vi "JKI SM Editor - Search String to Search Array.vi"(1 "String":string) -> (0 "Array":string[](array[string]))   [LabVIEW 2020]
uses:
  <userlib>/_OpenG.lib/string/string.llb/Trim Whitespace (String)__ogtk.vi
  <userlib>/_OpenG.lib/string/string.llb/openg_string.lvlib
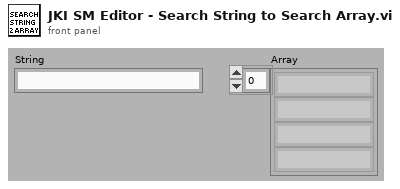
[diagram p1: front panel]
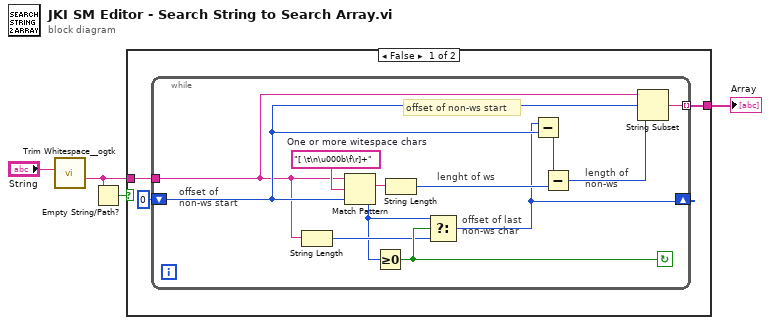
[diagram p0: block diagram]
diagram:
  n1 = call-poly <userlib>:"Trim Whitespace__ogtk.vi"("String in"="String") -> ("String out"=w2:string)  [unwired: 6 in]
  n2 = Empty String/Path?(string/path=w2) -> (empty?=w1:bool)
  n3 = case shown="False" w1 {
    tunnel: [w7 _] -> w4
    tunnel: w2 -> [w5 _]
    frame False {
      n4 = while {
        shift-right: [w8] -> _
        shift-left: 0 -> [w14]
        tunnel: w5 -> [w11]
        tunnel: [w15] -> w7 mode=indexing
        stop <- w12 continue-if-true
        w19 = "[ \t\n\u000b\f\r]+"  # One or more witespace chars
        # "offset of non-ws start"
        # "length of non-ws"
        # "offset of non-ws start"
        # "lenght of ws"
        # "offset of last non-ws char"
        n5 = String Length(string=w11) -> (length=w10:i32)
        n6 = Match Pattern(string=w11, regular expression=w19, offset (0)=w14) -> (match substring=w18:string, offset past match=w9:i32)  [unwired: 2 out]
        n7 = Greater Or Equal To 0?(x=w9) -> (x >= 0?=w12:bool)
        n8 = String Length(string=w18) -> (length=w17:i32)
        n9 = Select(t=w9, s=w12, f=w10) -> (s? t:f=w8:i32)
        n10 = Subtract(x=w8, y=w14) -> (x-y=w13:i32)
        n11 = Subtract(x=w13, y=w17) -> (x-y=w16:i32)
        n12 = String Subset(string=w11, offset (0)=w14, length (rest)=w16) -> (substring=w15:string)
      }
    }
    frame True {
    }
  }
  "Array" <- w4
